vi "Configure Digital Output.vi"(8 "error in (no error)":errorcluster, 10 "Digital Output (0)":i32 min=0 max=31 step=1, 11 "VISA resource name":refnum<visa-resource-name>) -> (0 "error out":errorcluster, 3 "VISA resource name out":refnum<visa-resource-name>)   [LabVIEW 2015, in "Lake Shore 372.lvlib"]
doc: "Configures the manual digital output settings using bit weighting. This function is only active if no Model 3726 Scanner is installed.\nBit: Weight: Name\n0 : 1 : D1\n1 : 2 : D2\n2 : 4 : D3\n3 : 8 : D4\n4 : 16 : D5"
uses:
  Lake Shore 372.lvlib
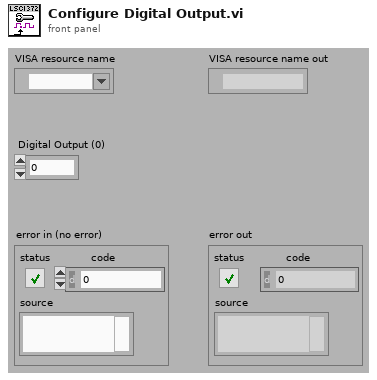
[diagram p1: front panel]
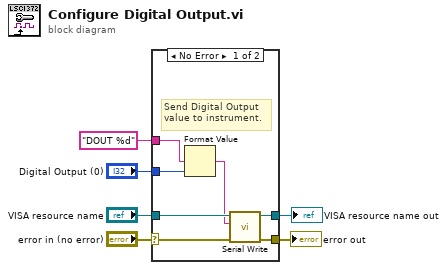
[diagram p0: block diagram]
diagram:
  n1 = case shown="No Error" "error in (no error)" {
    selector: "error in (no error)" -> [w7 w14]
    tunnel: "DOUT %d" -> [w13 _]
    tunnel: "Digital Output (0)" -> [w12 _]
    tunnel: "VISA resource name" -> [w11 w15]
    tunnel: [w10 w14] -> w3
    tunnel: [w9 w15] -> w2
    frame No Error {
      # "Send Digital Output\nvalue to instrument."
      n2 = Format Value(format string=w13, value (0)=w12) -> (output string=w8:string)  [unwired: 1 in]
      n3 = call "Serial Write.vi"("error in (no error)"=w7, "Write Buffer (\"\")"=w8, "VISA resource name"=w11) -> ("error out"=w10:errorcluster, "VISA resource name out"=w9:refnum<visa-resource-name>)  [unwired: 6 in, 1 out]
    }
    frame Error {
    }
  }
  "error out" <- w3
  "VISA resource name out" <- w2
